vi "Write UDP Connection Info.vi"(10 "connection info":T1, 11 "Wait On Assert ID in":refnum<class "Wait On Assert ID.lvclass">) -> (3 "Wait On Assert ID out":refnum<class "Wait On Assert ID.lvclass">)   [LabVIEW 2016, in "Assert API Components.lvlib" / "Assert Service.lvlib" / "Wait On Assert ID.lvclass"]
uses:
  Wait On Assert ID.lvclass
  <vilib>/NI/STM/UDP/UDP Connection Info.ctl
  <vilib>/NI/STM/SubVIs/MetaDataElement.ctl
  Wait On Assert ID.lvclass/Wait On Assert ID.ctl
  <vilib>/NI/STM/NI STM.lvlib
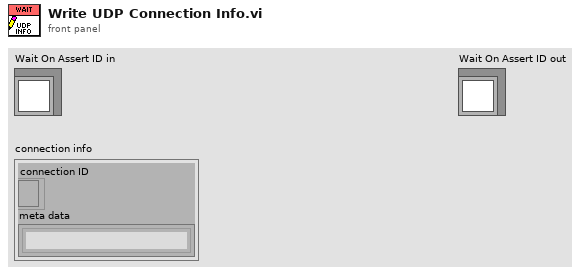
[diagram p1: front panel]
types:
  T1 = typedef "NI STM.lvlib/UDP Connection Info.ctl" = cluster{"connection ID":refnum<k16>, "meta data":T2[]}
  T2 = typedef "NI STM.lvlib/MetaDataElement.ctl" = string
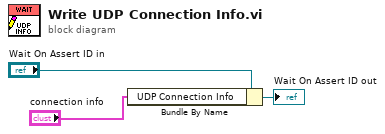
[diagram p0: block diagram]
diagram:
  n1 = Bundle By Name(cluster="Wait On Assert ID in", "UDP Connection Info"="connection info") -> (→"Wait On Assert ID out":refnum<class "Wait On Assert ID.lvclass">)
